vi "Expand Universe.vi"(11 "Univers In":string[][](array[string])) -> (1 "Expandable Columns":i32[](array[numeric]), 2 "Expandable Rows":i32[](array[numeric]), 3 "Universe Out":string[][](array[string]))   [LabVIEW 2021]
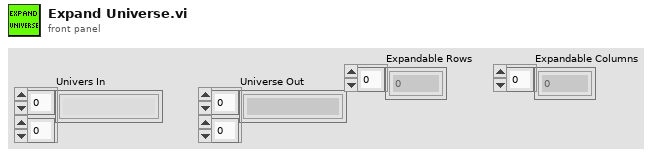
[diagram p1: front panel]
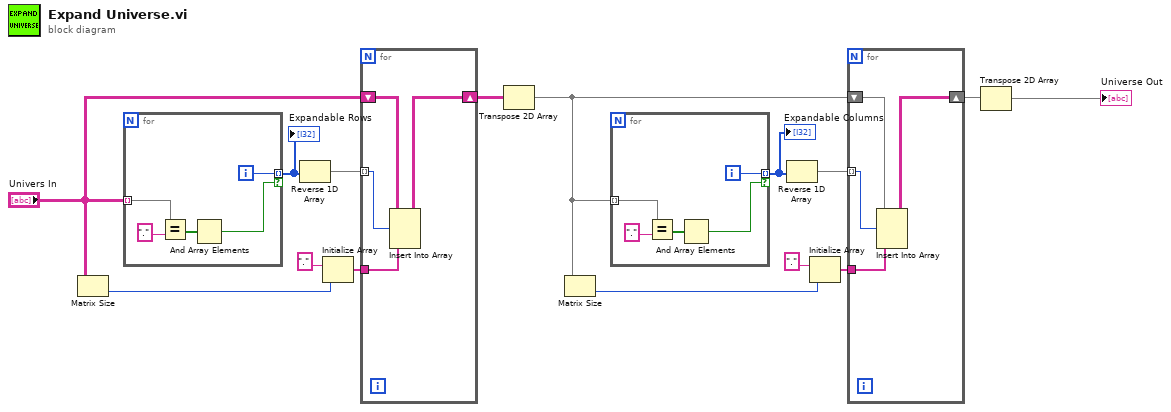
[diagram p0: block diagram]
diagram:
  n1 = Matrix Size(0:"Univers In") -> (2:w4:i32)  [unwired: 1 out]
  n2 = for {
    tunnel: "Univers In" -> [w20] mode=indexing
    tunnel: [w17] -> w1 mode=indexing if=w16
    i -> [w17]
    n3 = Equal?(x=w20, y=".") -> (x = y?=w18:bool[])
    n4 = And Array Elements(Boolean array=w18) -> (logical AND=w16:bool)
  }
  "Expandable Rows" <- w1
  n5 = Reverse 1D Array(array=w1) -> (reversed array=w7:i32[])
  n6 = Initialize Array(".", w4) -> (w5:string[])
  n7 = for {
    tunnel: w5 -> [w24]
    shift-right: [w21] -> w12
    shift-left: "Univers In" -> [w23]
    tunnel: w7 -> [w22] mode=indexing
    n8 = Insert Into Array(array=w23, index (row)=w22, new element=w24) -> (w21:string[][])  [unwired: 1 in]
  }
  n9 = Transpose 2D Array(2D array=w12) -> (transposed array=w13:string[][])
  n10 = Matrix Size(0:w13) -> (2:w10:i32)  [unwired: 1 out]
  n11 = for {
    tunnel: w13 -> [w29] mode=indexing
    tunnel: [w26] -> w2 mode=indexing if=w25
    i -> [w26]
    n12 = Equal?(x=w29, y=".") -> (x = y?=w27:bool[])
    n13 = And Array Elements(Boolean array=w27) -> (logical AND=w25:bool)
  }
  "Expandable Columns" <- w2
  n14 = Reverse 1D Array(array=w2) -> (reversed array=w8:i32[])
  n15 = Initialize Array(".", w10) -> (w9:string[])
  n16 = for {
    tunnel: w9 -> [w33]
    shift-right: [w30] -> w14
    shift-left: w13 -> [w32]
    tunnel: w8 -> [w31] mode=indexing
    n17 = Insert Into Array(array=w32, index (row)=w31, new element=w33) -> (w30:string[][])  [unwired: 1 in]
  }
  n18 = Transpose 2D Array(2D array=w14) -> (transposed array=→"Universe Out":string[][])
